vi "Populate Available Objects for PDO.vi"(8 "error in":errorcluster, 11 "UI Actor in":refnum<class "UI Actor.lvclass">) -> (0 "error out":errorcluster, 3 "UI Actor out":refnum<class "UI Actor.lvclass">)   [LabVIEW 2024, in "UI Actor.lvlib" / "UI Actor.lvclass"]
uses:
  UI Actor.lvclass
  UI Actor.lvclass/UI Actor.ctl
  Core/OD Entry/OD Entry.lvclass
  Core/EDS/EDS.lvclass
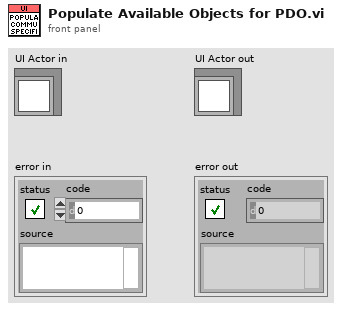
[diagram p1: front panel]
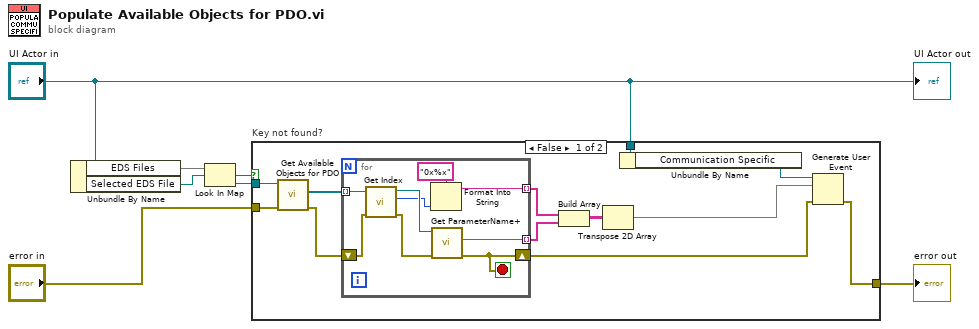
[diagram p0: block diagram]
diagram:
  n1 = Unbundle By Name("UI Actor in") -> ("EDS Files"=w7:map{path, refnum<class "EDS.lvclass">}, "Selected EDS File"=w6:path)
  n2 = Look In Map(map=w7, key=w6) -> (key not found?=w5:bool, value=w4:refnum<class "EDS.lvclass">)  [unwired: 1 in]
  n3 = case "Key not found?" shown="False" w5 {
    tunnel: w4 -> [w19 _]
    tunnel: "error in" -> [w18 w29]
    tunnel: [w8 w29] -> w1
    tunnel: "UI Actor in" -> [w14 _]
    frame False {
      n4 = call "Get Available Objects for PDO.vi"("error in"=w18, "EDS in"=w19) -> ("error out"=w16:errorcluster, "Entries"=w17:refnum<class "OD Entry.lvclass">[])  [unwired: 7 in, 1 out]
      n5 = for {
        tunnel: w17 -> [w28] mode=indexing
        tunnel: [w25] -> w10 mode=indexing
        shift-right: [w20] -> w9
        shift-left: w16 -> [w24]
        tunnel: [w21] -> w11 mode=indexing
        stop <- w20 stop-if-true
        n6 = call "Get Index.vi"("Error In"=w24, "reference in"=w28) -> ("Error Out"=w26:errorcluster, "Index"=w23:u16, "reference out"=w27:refnum<class "OD Entry.lvclass">)  [unwired: 7 in]
        n7 = Format Into String(format string="0x%x", w23) -> (resulting string=w21:string)  [unwired: 2 in, 1 out]
        n8 = call "Get ParameterName+.vi"("Error In"=w26, "reference in"=w27) -> ("Error Out"=w20:errorcluster, "ParameterName"=w25:string)  [unwired: 6 in, 2 out]
      }
      n9 = Build Array(w11, w10) -> (w12:string[][])
      n10 = Transpose 2D Array(2D array=w12) -> (transposed array=w13:string[][])
      n11 = Unbundle By Name(w14) -> ("Communication Specific"=w15:refnum<user-event>)
      n12 = Generate User Event(user event=w15, event data cluster=w13, error in=w9) -> (error out=w8:errorcluster)  [unwired: 1 in, 1 out]
    }
    frame True {
    }
  }
  "error out" <- w1
  "UI Actor out" <- "UI Actor in"
